vi "Custom_Profile_Dialog.vi"(11 "array":string[](array[string])) -> (2 "String":string, 3 "Cancelled?":bool)   [LabVIEW 2015]
doc: "Shows current profiles on the box for selection."
panel:
  in  "Profiles":i32(listbox)
  in  "Cancel":bool
  in  "OK":bool
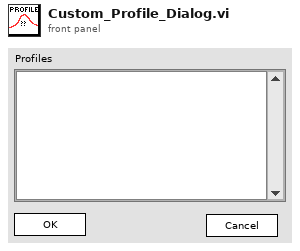
[diagram p1: front panel]
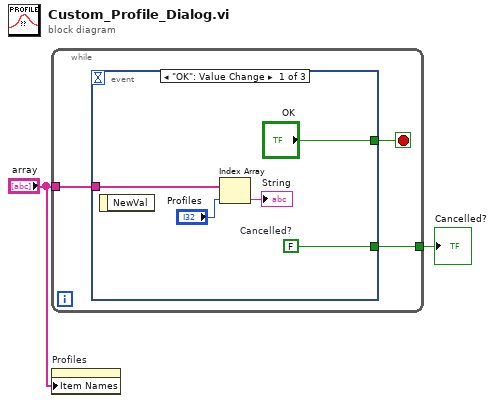
[diagram p0: block diagram]
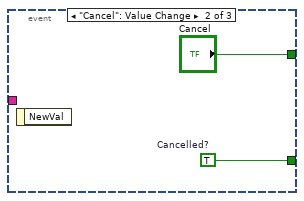
[diagram p2: hidden frame]
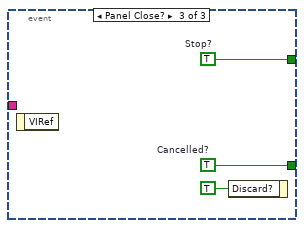
[diagram p3: hidden frame]
diagram:
  n1 = while {
    tunnel: [w4] -> w2
    tunnel: "array" -> [w3]
    stop <- w5 stop-if-true
    n2 = event shown="[0] \"OK\": Value Change" {
      selector: _ -> [_ _ _]
      dyn-events: _ -> [_ _ _]
      timeout: _ -> [_ _ _]
      tunnel: ["OK" "Cancel" w14] -> w5
      tunnel: [w10 w12 w13] -> w4
      tunnel: w3 -> [w6 _ _]
      event "OK": Value Change {
        w10 = FALSE  # Cancelled?
        n3 = event-data() -> ()  [unwired: 1 in, 1 out]
        n4 = Index Array(array=w6, index="Profiles") -> (element=→"String":string)
      }
      event "Cancel": Value Change {
        w12 = TRUE  # Cancelled?
        n5 = event-data() -> ()  [unwired: 1 in, 1 out]
      }
      event Panel Close? {
        w13 = TRUE  # Cancelled?
        w14 = TRUE  # Stop?
        n6 = event-data() -> ()  [unwired: 1 in, 1 out]
        n7 = event-data("Discard?"=TRUE) -> ()  [unwired: 1 in, 1 out]
      }
    }
  }
  "Cancelled?" <- w2
  n8 = property on="Profiles" class="LstBox (strict)"("Item Names"="array") -> ()  [unwired: 2 in, 2 out]
